vi "niSwitch Attach gRPC Session.vi"(8 "error in":errorcluster, 11 "resource name":string) -> (0 "error out":errorcluster, 3 "session factory out":refnum<class "Session Factory.lvclass">)   [LabVIEW 2021, in "Session Management niSwitch.lvlib" / "Session Factory.lvclass"]
doc: "Attaches to an existing session of the provided <b>resource name</b>."
uses:
  Session Factory.lvclass
  <vilib>/gRPC/Generated APIs/ni/measurementlink/discovery/v1/RPC Messages/ni_measurementlink_discovery_v1_ResolveServiceRequest.ctl
  <instrlib>/niSwitch/niSwitch.llb/niSwitch Topologies.ctl
  NI Switch Client/RPC Messages/niswitch_grpc_InitWithTopologyRequest.ctl
  NI Switch Client/RPC Messages/nidevice_grpc_SessionInitializationBehavior.ctl
  Session Factory.lvclass/Session Factory.ctl
  <vilib>/Plug-In SDKs/Clients/Discovery V1/NI Discovery V1 Client.lvlib
  NI Switch Client/NI Switch Client.lvlib
  <vilib>/gRPC/Generated APIs/ni/measurementlink/discovery/v1/ni.measurementlink.discovery.v1.api.lvlib
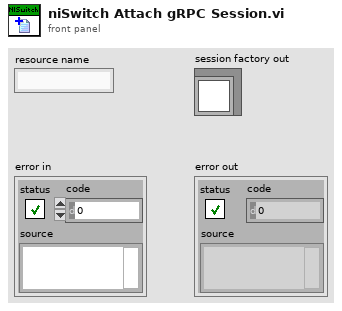
[diagram p1: front panel]
types:
  T1 = typedef "NI Switch Client.lvlib/nidevice_grpc_SessionInitializationBehavior.ctl" = enum32{"SESSION_INITIALIZATION_BEHAVIOR_UNSPECIFIED", "SESSION_INITIALIZATION_BEHAVIOR_INITIALIZE_NEW", "SESSION_INITIALIZATION_BEHAVIOR_ATTACH_TO_EXISTING"}
  T2 = typedef "NI Switch Client.lvlib/niswitch_grpc_InitWithTopologyRequest.ctl" = cluster{"session_name":string, "resource_name":string, "topology":string, "simulate":bool, "reset_device":bool, "initialization_behavior":T1}
  T3 = typedef "niSwitch Topologies.ctl" = string
  T4 = typedef "ni.measurementlink.discovery.v1.api.lvlib/ni_measurementlink_discovery_v1_ResolveServiceRequest.ctl" = cluster{"provided_interface":string, "service_class":string, "deployment_target":string, "version":string}
  T5 = typedef "ni.measurementlink.discovery.v1.api.lvlib/ni_measurementlink_discovery_v1_ServiceLocation.ctl" = cluster{"location":string, "insecure_port":string, "ssl_authenticated_port":string}
  T6 = typedef "grpc-lvsupport-release.lvlib/grpcId.ctl" = u64
  T7 = typedef "NI Switch Client.lvlib/niswitch_grpc_InitWithTopologyResponse.ctl" = cluster{"status":i32, "vi":T8, "error_message":string, "new_session_initialized":bool}
  T8 = typedef "NI Switch Client.lvlib/nidevice_grpc_Session.ctl" = cluster{"nidevice_grpc_Session_session":refnum<class "nidevice_grpc_Session_session.lvclass">}
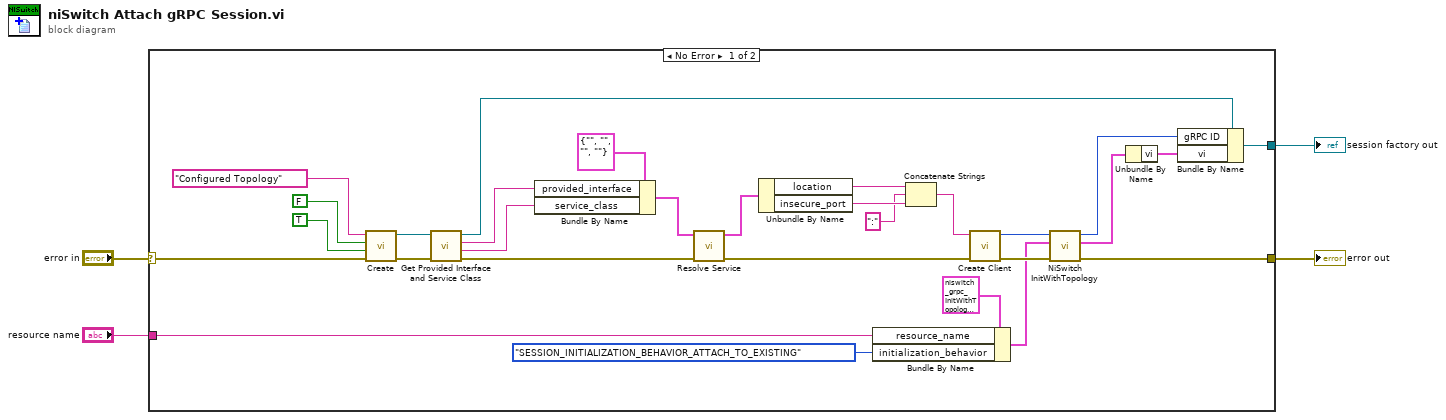
[diagram p0: block diagram]
diagram:
  n1 = case shown="No Error" "error in" {
    selector: "error in" -> [w32 w34]
    tunnel: "resource name" -> [w8 _]
    tunnel: [w18 w34] -> w2
    tunnel: [w10 _] -> w1
    frame No Error {
      n2 = call "Create.vi"("error in"=w32, "reset device"=TRUE, "simulate"=FALSE, "topology name"=T3 "Configured Topology") -> ("error out"=w33:errorcluster, "session factory out"=w5:refnum<class "Session Factory.lvclass">)  [unwired: 6 in]
      n3 = call-dynamic "Get Provided Interface and Service Class.vi"("error in"=w33, "session factory in"=w5) -> ("error out"=w23:errorcluster, "service class"=w22:string, "provided interface"=w21:string, "session factory out"=w7:refnum<class "Session Factory.lvclass">)  [unwired: 6 in]
      n4 = Bundle By Name(cluster=T4 {"provided_interface"="", "service_class"="", "deployment_target"="", "version"=""} ("request data"), "provided_interface"=w21, "service_class"=w22) -> (w14:T4)
      n5 = call <vilib>:"Resolve Service.vi"("error in"=w23, "request data"=w14) -> ("error out"=w26:errorcluster, "response data"=w15:T5)  [unwired: 8 in]
      n6 = Unbundle By Name(w15) -> ("location"=w12:string, "insecure_port"=w13:string)
      n7 = Bundle By Name(cluster=T2 {"session_name"="", "resource_name"="", "topology"="", "simulate"=FALSE, "reset_device"=FALSE, "initialization_behavior"=enum."SESSION_INITIALIZATION_BEHAVIOR_UNSPECIFIED"} ("Request Data"), "resource_name"=w8, "initialization_behavior"=nidevice_grpc_SessionInitializationBehavior."SESSION_INITIALIZATION_BEHAVIOR_ATTACH_TO_EXISTING") -> (w19:T2)
      n8 = Concatenate Strings(w12, ":" ("string"), w13) -> (w27:string)
      n9 = call "Create Client.vi"("error in"=w26, "address"=w27) -> ("error out"=w25:errorcluster, "gRPC ID Out"=w24:T6)  [unwired: 8 in]
      n10 = call "NiSwitch InitWithTopology.vi"("error in"=w25, "Request Data"=w19, "gRPC ID"=w24) -> ("error out"=w18:errorcluster, "Response Data"=w6:T7, "gRPC ID out"=w17:T6)  [unwired: 6 in]
      n11 = Unbundle By Name(w6) -> ("vi"=w16:T8)
      n12 = Bundle By Name(cluster=w7, "gRPC ID"=w17, "vi"=w16) -> (w10:refnum<class "Session Factory.lvclass">)
    }
    frame Error {
    }
  }
  "error out" <- w2
  "session factory out" <- w1
